vi "AddCursor.vi"(7 "LabVIEW Web Service Request":refnum<class "Web Request.lvclass">) -> (3 "value":string)   [LabVIEW 2014]
uses:
  <vilib>/wsapi/Web Request.lvclass
  Libraries/Map Data Folder/CursorList.ctl
  Libraries/Map Data Folder/Map Data.lvlib
panel:
  out "rest of the binary string":string
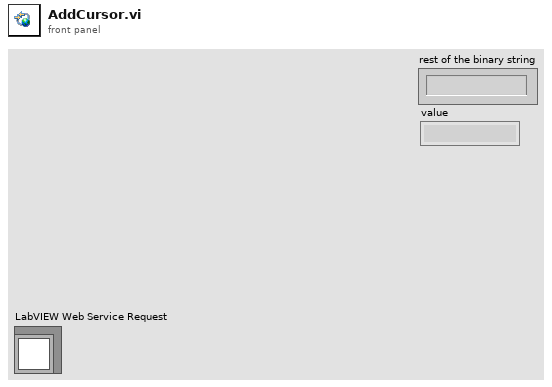
[diagram p1: front panel]
types:
  T1 = typedef "Map Data.lvlib/CursorList.ctl" = cluster{"Name":string, "Color":u32, "Style":u8, "Point Style":u8, "Name Visible":bool, "Allow Drag":bool, "Cursor Mode":u32, "Plot":i32, "Index":i32, "Position":cluster{"X":dbl, "Y":dbl}, "X Scale":u32, "Y Scale":u32, "Watch Plots":i32[], "Watch All Plots":bool, "Plot Area":i32, "Label Offset":cluster{"X":dbl, "Y":dbl}}[]
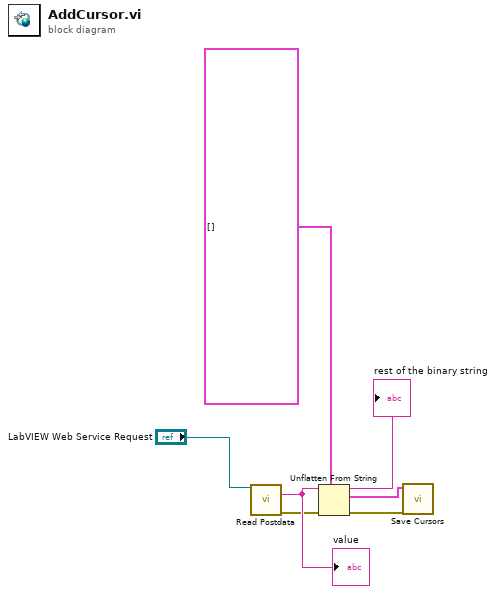
[diagram p0: block diagram]
diagram:
  n1 = call <vilib>:"Read Postdata.vi"("LabVIEW Web Service Request"="LabVIEW Web Service Request") -> ("postdata"=w4:string, "error out"=w3:errorcluster)  [unwired: 12 in, 1 out]
  "value" <- w4
  n2 = Unflatten From String(type=T1 [] ("Cursor List"), binary string=w4, error in (no error)=w3) -> (rest of the binary string=→"rest of the binary string":string, value=w1:T1, error out=w6:errorcluster)  [unwired: 2 in]
  n3 = call "Save Cursors.vi"("error in (no error)"=w6, "Cursor List"=w1) -> ()  [unwired: 8 in, 2 out]
